vi "Exporting.vi"() -> ()   [LabVIEW 2010]
uses:
  C:/Program Files/Spiricon/BeamGage Enterprise/Spiricon.BeamGage.Automation.Interfaces.dll
  Program Files/Spiricon/BeamGage Enterprise/Spiricon.BeamGage.Automation.Interfaces.dll
  C:/Program Files/Spiricon/BeamGage Enterprise/Spiricon.BeamGage.Automation.dll
  Program Files/Spiricon/BeamGage Enterprise/Spiricon.BeamGage.Automation.dll
panel:
  out "Callback2Exists":bool
  out "Callback1Exists":bool
  in  "STOP SERVER":bool
  in  "START_STOP":bool
  out "AExportStatusEnum":T1(ring)
  in  "EXPORT IMAGE":bool
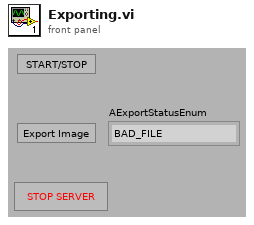
[diagram p1: front panel]
types:
  T1 = enum16{"BAD_FILE", "BAD_FRAME_NUM", "BASE_FILE_EXISTS", "BASE_FILE_IS_DIRECTORY", "GOOD", "NO_FILE_NAME", "NO_IMAGE", "READ_ONLY", "null"}
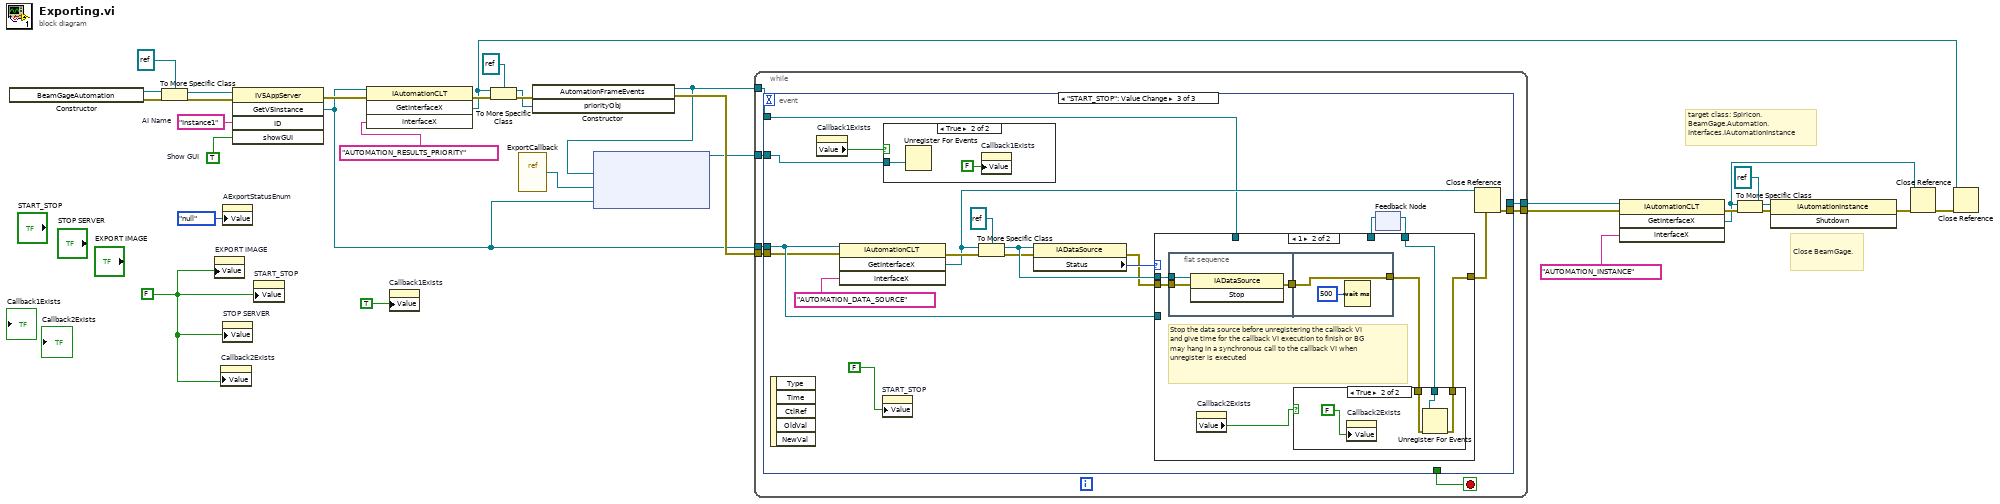
[diagram p0: block diagram]
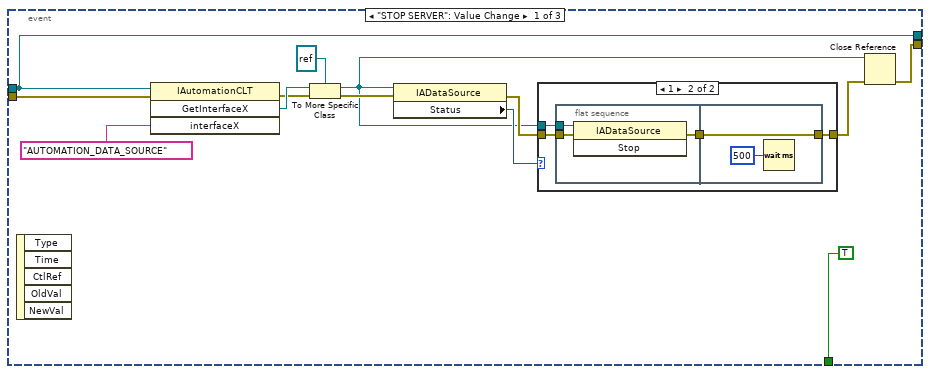
[diagram p2: hidden frame]
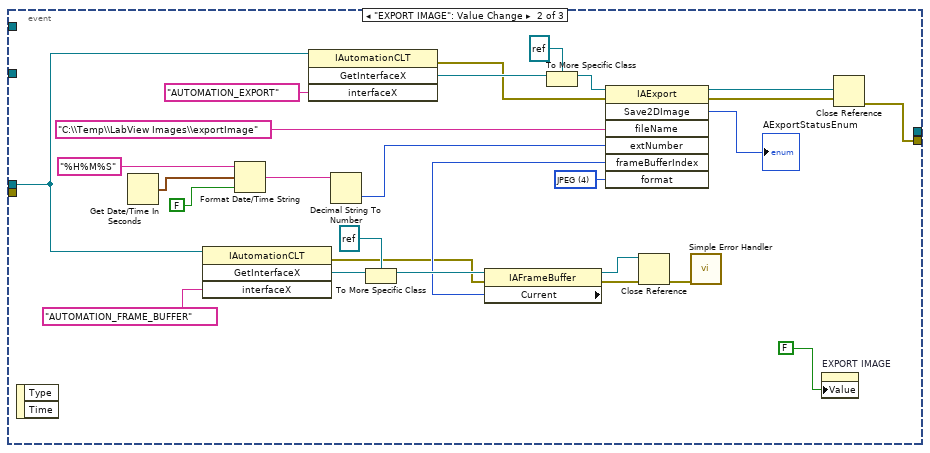
[diagram p4: hidden frame]
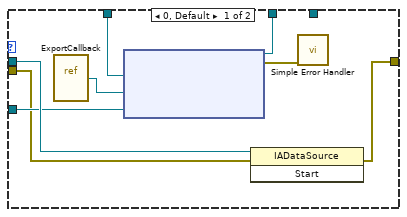
[diagram p6: hidden frame]
diagram:
  w20 = TRUE  # Show GUI
  w24 = "Instance1"  # AI Name
  w3 = FALSE ("stop")
  # "Close BeamGage."
  # "target class: Spiricon.BeamGage.Automation.Interfaces.IAutomationInstance"
  n1 = constructor class="BeamGageAutomation"() -> (reference out=w21:refnum<k24>, error out=w28:errorcluster)  [unwired: 3 in, 1 out]
  n2 = To More Specific Class(target class=refnum<k24> refnum, reference=w21, error in=w28) -> (specific class reference=w26:refnum<k24>, error out=w27:errorcluster)
  n3 = property on="EXPORT IMAGE" class="Bool (strict)"("Value"=w3) -> ()  [unwired: 2 in, 2 out]
  n4 = property on="Callback2Exists" class="Bool (strict)"("Value"=w3) -> ()  [unwired: 2 in, 2 out]
  n5 = property on="AExportStatusEnum" class="Enum (strict)"("Value"=T1."null" ("AExportStatusEnum")) -> ()  [unwired: 2 in, 2 out]
  n6 = property on="STOP SERVER" class="Bool (strict)"("Value"=w3) -> ()  [unwired: 2 in, 2 out]
  n7 = invoke class="IV5AppServer" method="GetV5Instance"(reference=w26, error in=w27, "ID"=w24, "showGUI"=w20) -> (error out=w25:errorcluster, "GetV5Instance"=w5:refnum<k24>)  [unwired: 1 in, 3 out]
  n8 = property on="START_STOP" class="Bool (strict)"("Value"=w3) -> ()  [unwired: 2 in, 2 out]
  n9 = invoke class="IAutomationCLT" method="GetInterfaceX"(reference=w5, error in=w25, "interfaceX"="AUTOMATION_RESULTS_PRIORITY") -> (error out=w31:errorcluster, "GetInterfaceX"=w1:refnum<k24>)  [unwired: 1 in, 2 out]
  n10 = property on="Callback1Exists" class="Bool (strict)"("Value"=TRUE ("CallbackExists")) -> ()  [unwired: 2 in, 2 out]
  n11 = To More Specific Class(target class=refnum<k24> refnum, reference=w1, error in=w31) -> (specific class reference=w22:refnum<k24>, error out=w32:errorcluster)
  n12 = vi-ref "ExportCallback.vi"() -> ("vi reference"=w8:refnum<vi>)
  n13 = constructor class="AutomationFrameEvents"(error in=w32, "priorityObj"=w22) -> (reference out=w6:refnum<k24>, error out=w10:errorcluster)  [unwired: 2 in, 2 out]
  n14 = node(w6, w8, w5) -> (w7:refnum<k27>)  [unwired: 2 in, 1 out]
  n15 = while {
    tunnel: [w39] -> w12
    tunnel: w5 -> [w35]
    tunnel: w10 -> [w37]
    tunnel: [w36] -> w11
    tunnel: w6 -> [w34]
    tunnel: w7 -> [w33]
    stop <- w38 stop-if-true
    n16 = event shown="[2] \"START_STOP\": Value Change" {
      selector: _ -> [_ _ _]
      dyn-events: _ -> [_ _ _]
      timeout: _ -> [_ _ _]
      tunnel: [w40 _ _] -> w39
      tunnel: [TRUE ("stop") _ _] -> w38
      tunnel: w37 -> [w43 _ w93]
      tunnel: [w44 w66 w94] -> w36
      tunnel: w35 -> [w40 w69 w95]
      tunnel: w34 -> [_ _ w97]
      tunnel: w33 -> [_ _ w91]
      event "STOP SERVER": Value Change {
        n17 = event-data() -> ()  [unwired: 1 in, 5 out]
        n18 = invoke class="IAutomationCLT" method="GetInterfaceX"(reference=w40, error in=w43, "interfaceX"="AUTOMATION_DATA_SOURCE") -> (error out=w48:errorcluster, "GetInterfaceX"=w51:refnum<k24>)  [unwired: 1 in, 2 out]
        n19 = To More Specific Class(target class=refnum<k24> refnum, reference=w51, error in=w48) -> (specific class reference=w41:refnum<k24>, error out=w46:errorcluster)
        n20 = property class="IADataSource"(reference=w41, error in=w46) -> (error out=w49:errorcluster, "Status"=w45:i32)  [unwired: 1 out]
        n21 = case shown="1" w45 {
          tunnel: w41 -> [_ w57]
          tunnel: w49 -> [w53 w56]
          tunnel: [w53 w55] -> w50
          frame 0, Default {
          }
          frame 1 {
            n22 = flat-sequence {
              tunnel: w57 -> [w60]
              tunnel: w56 -> [w59]
              tunnel: [w58] -> w54
              tunnel: [w61] -> w55
              tunnel: w54 -> [w61]
              frame #0 {
                n23 = invoke class="IADataSource" method="Stop"(reference=w60, error in=w59) -> (error out=w58:errorcluster)  [unwired: 1 in, 2 out]
              }
              frame #1 {
                n24 = Wait (ms)(milliseconds to wait=u32 500) -> ()  [unwired: 1 out]
              }
            }
          }
        }
        n25 = Close Reference(reference=w41, error in (no error)=w50) -> (error out=w44:errorcluster)
      }
      event "EXPORT IMAGE": Value Change {
        w80 = 4 items=["NONE", "ASCII", "BMP", "GIF", "JPEG", "PNG", "TIFF"] ("format")
        n26 = event-data() -> ()  [unwired: 1 in, 2 out]
        n27 = Get Date/Time In Seconds() -> (seconds since 1Jan1904=w87:timestamp)
        n28 = invoke class="IAutomationCLT" method="GetInterfaceX"(reference=w69, "interfaceX"="AUTOMATION_FRAME_BUFFER") -> (error out=w67:errorcluster, "GetInterfaceX"=w74:refnum<k24>)  [unwired: 2 in, 2 out]
        n29 = Format Date/Time String(time format string (%c)="%H%M%S", seconds (now)=w87, UTC format=FALSE) -> (date/time string=w83:string)
        n30 = invoke class="IAutomationCLT" method="GetInterfaceX"(reference=w69, "interfaceX"="AUTOMATION_EXPORT") -> (error out=w68:errorcluster, "GetInterfaceX"=w77:refnum<k24>)  [unwired: 2 in, 2 out]
        n31 = Decimal String To Number(string=w83) -> (number=w84:i32)  [unwired: 2 in, 1 out]
        n32 = To More Specific Class(target class=refnum<k24> refnum, reference=w74) -> (specific class reference=w72:refnum<k24>)  [unwired: 1 in, 1 out]
        n33 = property class="IAFrameBuffer"(reference=w72, error in=w67) -> (reference out=w63:refnum<k24>, error out=w64:errorcluster, "Current"=w71:u32)
        n34 = To More Specific Class(target class=refnum<k24> refnum, reference=w77) -> (specific class reference=w88:refnum<k24>)  [unwired: 1 in, 1 out]
        n35 = invoke class="IAExport" method="Save2DImage"(reference=w88, error in=w68, "fileName"="C:\\Temp\\LabView Images\\exportImage", "extNumber"=w84, "frameBufferIndex"=w71, "format"=w80) -> (reference out=w82:refnum<k24>, error out=w81:errorcluster, "Save2DImage"=→"AExportStatusEnum":i32)  [unwired: 1 in, 4 out]
        n36 = Close Reference(reference=w63, error in (no error)=w64) -> (error out=w65:errorcluster)
        n37 = call <vilib>:"Simple Error Handler.vi"("error in (no error)"=w65) -> ()  [unwired: 4 in, 5 out]
        n38 = property on="EXPORT IMAGE" class="Bool (strict)"("Value"=FALSE ("stop")) -> ()  [unwired: 2 in, 2 out]
        n39 = Close Reference(reference=w82, error in (no error)=w81) -> (error out=w66:errorcluster)
      }
      event "START_STOP": Value Change {
        n40 = event-data() -> ()  [unwired: 1 in, 5 out]
        n41 = property on="Callback1Exists" class="Bool (strict)"() -> ("Value"=w90:bool)  [unwired: 2 in, 2 out]
        n42 = invoke class="IAutomationCLT" method="GetInterfaceX"(reference=w95, error in=w93, "interfaceX"="AUTOMATION_DATA_SOURCE") -> (error out=w102:errorcluster, "GetInterfaceX"=w98:refnum<k24>)  [unwired: 1 in, 2 out]
        n43 = property on="START_STOP" class="Bool (strict)"("Value"=FALSE ("stop")) -> ()  [unwired: 2 in, 2 out]
        n44 = case shown="True" w90 {
          tunnel: w91 -> [_ w109]
          frame False {
          }
          frame True {
            n45 = Unregister For Events(event registration refnum=w109) -> ()  [unwired: 1 in, 1 out]
            n46 = property on="Callback1Exists" class="Bool (strict)"("Value"=FALSE ("CallbackExists")) -> ()  [unwired: 2 in, 2 out]
          }
        }
        n47 = To More Specific Class(target class=refnum<k24> refnum, reference=w98, error in=w102) -> (specific class reference=w107:refnum<k24>, error out=w105:errorcluster)
        n48 = property class="IADataSource"(reference=w107, error in=w105) -> (error out=w101:errorcluster, "Status"=w106:i32)  [unwired: 1 out]
        n49 = feedback #1() -> (w92:refnum<k27>)  [unwired: 1 in]
        n50 = case shown="1" w106 {
          tunnel: w107 -> [w117 w123]
          tunnel: w101 -> [w110 w122]
          tunnel: [w116 w119] -> w99
          tunnel: [w115 _] -> w96
          tunnel: w97 -> [w112 _]
          tunnel: w92 -> [_ w121]
          tunnel: w95 -> [w113 _]
          frame 0, Default {
            n51 = vi-ref "ExportCallback.vi"() -> ("vi reference"=w114:refnum<vi>)
            n52 = node(w112, w114, w113) -> (w115:refnum<k27>, w111:errorcluster)  [unwired: 2 in]
            n53 = invoke class="IADataSource" method="Start"(reference=w117, error in=w110) -> (error out=w116:errorcluster)  [unwired: 1 in, 2 out]
            n54 = call <vilib>:"Simple Error Handler.vi"("error in (no error)"=w111) -> ()  [unwired: 4 in, 5 out]
          }
          frame 1 {
            # "Stop the data source before unregistering the callback VI  and give time for the callback VI execution to finish or BG may hang in a synchronous call to the callback VI when unregister is executed"
            n55 = flat-sequence {
              tunnel: w123 -> [w131]
              tunnel: w122 -> [w130]
              tunnel: [w129] -> w124
              tunnel: [w132] -> w120
              tunnel: w124 -> [w132]
              frame #0 {
                n56 = invoke class="IADataSource" method="Stop"(reference=w131, error in=w130) -> (error out=w129:errorcluster)  [unwired: 1 in, 2 out]
              }
              frame #1 {
                n57 = Wait (ms)(milliseconds to wait=u32 500) -> ()  [unwired: 1 out]
              }
            }
            n58 = property on="Callback2Exists" class="Bool (strict)"() -> ("Value"=w118:bool)  [unwired: 2 in, 2 out]
            n59 = case shown="True" w118 {
              tunnel: w121 -> [_ w128]
              tunnel: w120 -> [_ w126]
              tunnel: [_ w125] -> w119
              frame False {
              }
              frame True {
                n60 = property on="Callback2Exists" class="Bool (strict)"("Value"=FALSE ("CallbackExists")) -> ()  [unwired: 2 in, 2 out]
                n61 = Unregister For Events(event registration refnum=w128, error in=w126) -> (error out=w125:errorcluster)
              }
            }
          }
        }
        n62 = feedback-in #1(w96) -> ()
        n63 = Close Reference(reference=w98, error in (no error)=w99) -> (error out=w94:errorcluster)
      }
    }
  }
  n64 = invoke class="IAutomationCLT" method="GetInterfaceX"(reference=w12, error in=w11, "interfaceX"="AUTOMATION_INSTANCE") -> (error out=w15:errorcluster, "GetInterfaceX"=w13:refnum<k24>)  [unwired: 1 in, 2 out]
  n65 = To More Specific Class(target class=refnum<k24> refnum, reference=w13, error in=w15) -> (specific class reference=w16:refnum<k24>, error out=w14:errorcluster)
  n66 = invoke class="IAutomationInstance" method="Shutdown"(reference=w16, error in=w14) -> (error out=w19:errorcluster)  [unwired: 1 in, 2 out]
  n67 = Close Reference(reference=w13, error in (no error)=w19) -> (error out=w2:errorcluster)
  n68 = Close Reference(reference=w1, error in (no error)=w2) -> ()  [unwired: 1 out]
